vi "Acquisition_1channel.vi"() -> ()   [LabVIEW 2014]
uses:
  <vilib>/rvi/Emulation/niFpgaGetClockAttributes.vi
  <vilib>/rvi/Emulation/niFpgaSctlEmulationGetInTimedLoop.vi
  <vilib>/rvi/Emulation/niFpgaEmulationReportErrorSimple.vi
  <vilib>/rvi/eio/common/nirviEmuTemplateMethod_errors.vi
  <vilib>/rvi/interface/RandomDataEmulation/niFpgaRandomDataHandleErrors.vi
  <vilib>/rvi/Emulation/niFpgaCriticalErrorInLSC.vi
  <vilib>/eio/EIONode/EIONode.xnode
  <vilib>/rvi/DataTransferAndStorage/Container/XNode/niFpgaContainer.xnode
  <vilib>/rvi/interface/RandomDataEmulation/nirviRandomDataFpgaReadWriteTemplate.vi
panel:
  out "FIFO timeout":bool
  out "Connector0/AI6":i16
  out "Acquisition\nTimeout":bool
  in  "Sampling(Ticks)":u32 caption="Count(Ticks)"
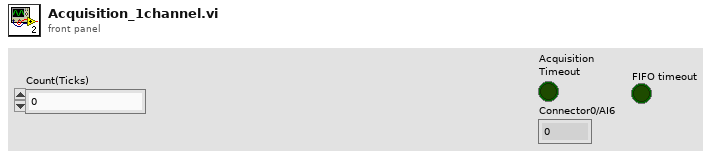
[diagram p1: front panel]
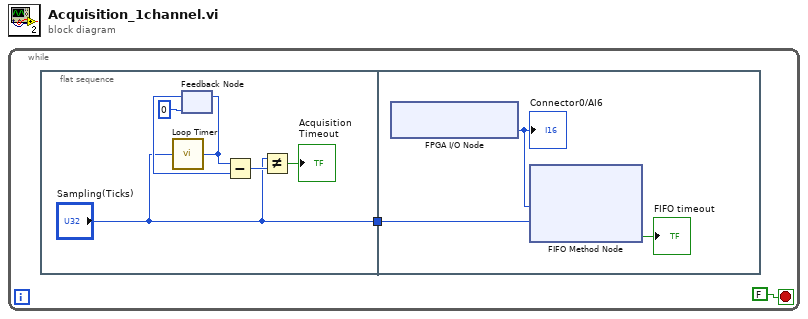
[diagram p0: block diagram]
diagram:
  n1 = while {
    stop <- FALSE stop-if-true
    n2 = flat-sequence {
      tunnel: ["Sampling(Ticks)"] -> w1
      tunnel: w1 -> [w10]
      frame #0 {
        n3 = call "Loop Timer"("Count(Ticks)"="Sampling(Ticks)") -> ("Tick Count(Ticks)"=w7:u32)
        n4 = feedback-in #1(w7) -> ()
        n5 = feedback #1(u32 0 ("Tick Count(Ticks)")) -> (w6:u32)
        n6 = Subtract(x=w7, y=w6) -> (x-y=w5:u32)
        n7 = Not Equal?(x="Sampling(Ticks)", y=w5) -> (x != y?=→"Acquisition\nTimeout":bool)
      }
      frame #1 {
        n8 = xnode "FPGA I/O Node"() -> ("Connector0/AI6"=w11:i16)  [unwired: 1 in, 1 out]
        "Connector0/AI6" <- w11
        n9 = xnode ("FIFO Method Node")("Element"=w11, "Timeout"=w10) -> ("Timed Out?"=→"FIFO timeout":bool)  [unwired: 1 in, 1 out]
      }
    }
  }
